vi "Read EMS Message.vi"(11 "EMS Message Msg in":refnum<class "EMS Message Msg.lvclass">) -> (2 "Message":T1, 3 "EMS Message Msg out":refnum<class "EMS Message Msg.lvclass">)   [LabVIEW 2015, in "SCADA Communcations Actor.lvlib" / "EMS Message Msg.lvclass"]
uses:
  EMS Message Msg.lvclass
  SCADA Communications/Controls/EMS Message Cluster.ctl
  EMS Message Msg.lvclass/EMS Message Msg.ctl
  SCADA Communications/SCADA Communications.lvclass
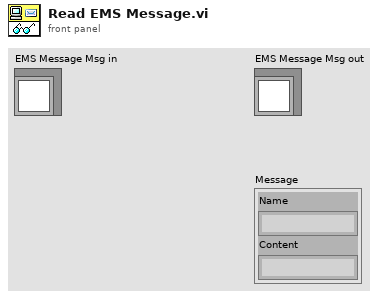
[diagram p1: front panel]
types:
  T1 = typedef "SCADA Communcations Actor.lvlib/SCADA Communications.lvclass/EMS Message Cluster.ctl" = cluster{"Name":string, "Content":string}
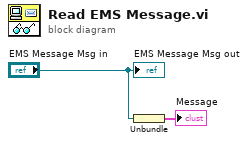
[diagram p0: block diagram]
diagram:
  n1 = Unbundle("EMS Message Msg in") -> (→"Message":T1)
  "EMS Message Msg out" <- "EMS Message Msg in"
